vi "CameraTest.vi"() -> ()   [LabVIEW 2016]
uses:
  <vilib>/userdefined/High Color/IMAQdx.ctl
  ListboxMenu/listbox/listbox.lvclass
  ListboxMenu/listbox/listbox.lvclass/listbox.ctl
  ListboxMenu/LNK/UP/UP.lvclass
  C:/Users/ok/Desktop/camera parameters/ListboxMenu/LNK/Parent Class/Menu.lvclass
  ListboxMenu/LNK/Delete/Delete.lvclass
  ListboxMenu/LNK/Down/Down.lvclass
  <vilib>/Utility/miscctls.llb/LVRowAndColumnTypeDef.ctl
  <vilib>/Utility/miscctls.llb/LVPositionTypeDef.ctl
  <vilib>/vision/driver/NI_Vision_Acquisition_Software.lvlib
  <resource>/objmgr/imaqdx.rc
  <vilib>/ptbypt/NI_PtbyPt.lvlib
panel:
  in  "搜索相机":bool
  in  "启动相机":bool
  in  "停止相机":bool
  in  "连续获取":bool
  in  "单次获取":bool
  out "Image":T1(plugin-control)
  in  "Enum":u16(ring) items=["Off", "On"]
  in  "String":string
  in  "U32":i16
  in  "I64":i64
  in  "DBL":dbl
  in  "Bool":bool
  in  "写入参数文件":bool
  in  "读取参数文件":bool
  in  "相机参数列表":u16(ring) items=["NULL", "AcquisitionAttributes::AdvancedEthernet::BandwidthControl::DesiredPeakBandwidth", "AcquisitionAttributes::AdvancedEthernet::Controller::DestinationMode", "AcquisitionAttributes::AdvancedEthernet::Controller::DestinationMulticastAddress", "AcquisitionAttributes::AdvancedEthernet::EventParameters::MaxOutstandingEvents", "AcquisitionAttributes::AdvancedEthernet::FirewallTraversal::Enabled", "AcquisitionAttributes::AdvancedEthernet::FirewallTraversal::KeepAliveTime", "AcquisitionAttributes::AdvancedEthernet::ResendParameters::MaxResendsPerPacket", "AcquisitionAttributes::AdvancedEthernet::ResendParameters::MemoryWindowSize", "AcquisitionAttributes::AdvancedEthernet::ResendParameters::MissingPacketTimeout", "AcquisitionAttributes::AdvancedEthernet::ResendParameters::NewPacketTimeout", "AcquisitionAttributes::AdvancedEthernet::ResendParameters::ResendBatchingPercentage", "AcquisitionAttributes::AdvancedEthernet::ResendParameters::ResendResponseTimeout", "AcquisitionAttributes::AdvancedEthernet::ResendParameters::ResendThresholdPercentage", "AcquisitionAttributes::AdvancedEthernet::ResendParameters::ResendTimerResolution", "AcquisitionAttributes::AdvancedEthernet::ResendParameters::ResendsEnabled", "AcquisitionAttributes::AdvancedEthernet::TestPacketParameters::MaxTestPacketRetries", "AcquisitionAttributes::AdvancedEthernet::TestPacketParameters::TestPacketEnabled", "AcquisitionAttributes::AdvancedEthernet::TestPacketParameters::TestPacketTimeout", "AcquisitionAttributes::AdvancedGenicam::CommandTimeout", "AcquisitionAttributes::AdvancedGenicam::EventsEnabled", "AcquisitionAttributes::AdvancedGenicam::IgnoreCameraValidationErrors", "AcquisitionAttributes::Bayer::Algorithm", "AcquisitionAttributes::Bayer::GainB", "AcquisitionAttributes::Bayer::GainG", "AcquisitionAttributes::Bayer::GainR", "AcquisitionAttributes::Bayer::Pattern", "AcquisitionAttributes::ChunkDataDecoding::ChunkDataDecodingEnabled", "AcquisitionAttributes::ChunkDataDecoding::MaximumChunkCopySize", "CameraAttributes::AnalogControls::GainAuto", "CameraAttributes::AnalogControls::GainSelector", "CameraAttributes::AnalogControls::GainRaw", "CameraAttributes::AnalogControls::BlackLevelSelector", "CameraAttributes::AnalogControls::BlackLevelRaw", "CameraAttributes::AnalogControls::GammaEnable", "CameraAttributes::AnalogControls::GammaSelector", "CameraAttributes::AnalogControls::Gamma", "CameraAttributes::AnalogControls::DigitalShift", "CameraAttributes::ImageFormat::PixelFormat", "CameraAttributes::ImageFormat::ReverseX", "CameraAttributes::ImageFormat::TestImageSelector", "CameraAttributes::AOI::Width", "CameraAttributes::AOI::Height", "CameraAttributes::AOI::OffsetX", "CameraAttributes::AOI::OffsetY", "CameraAttributes::AOI::CenterX", "CameraAttributes::AOI::CenterY", "CameraAttributes::AOI::BinningHorizontal", "CameraAttributes::AOI::BinningVertical", "CameraAttributes::AcquisitionTrigger::AcquisitionMode", "CameraAttributes::AcquisitionTrigger::AcquisitionFrameCount", "CameraAttributes::AcquisitionTrigger::TriggerSelector", "CameraAttributes::AcquisitionTrigger::TriggerMode", "CameraAttributes::AcquisitionTrigger::TriggerSoftware", "CameraAttributes::AcquisitionTrigger::TriggerSource", "CameraAttributes::AcquisitionTrigger::TriggerActivation", "CameraAttributes::AcquisitionTrigger::TriggerDelayAbs", "CameraAttributes::AcquisitionTrigger::ExposureMode", "CameraAttributes::AcquisitionTrigger::ExposureAuto", "CameraAttributes::AcquisitionTrigger::ExposureTimeAbs", "CameraAttributes::AcquisitionTrigger::ExposureTimeRaw", "CameraAttributes::AcquisitionTrigger::GlobalResetReleaseModeEnable", "CameraAttributes::AcquisitionTrigger::AcquisitionFrameRateEnable", "CameraAttributes::AcquisitionTrigger::AcquisitionFrameRateAbs", "CameraAttributes::AcquisitionTrigger::AcquisitionStatusSelector", "CameraAttributes::DigitalIO::LineSelector", "CameraAttributes::DigitalIO::LineMode", "CameraAttributes::DigitalIO::LineFormat", "CameraAttributes::DigitalIO::LineSource", "CameraAttributes::DigitalIO::LineInverter", "CameraAttributes::DigitalIO::UserOutputSelector", "CameraAttributes::DigitalIO::UserOutputValue", "CameraAttributes::DigitalIO::UserOutputValueAll", "CameraAttributes::SequenceControl::SequenceEnable", "CameraAttributes::SequenceControl::SequenceControlConfiguration::SequenceAdvanceMode", "CameraAttributes::SequenceControl::SequenceSetTotalNumber", "CameraAttributes::SequenceControl::SequenceSetIndex", "CameraAttributes::SequenceControl::SequenceSetStore", "CameraAttributes::SequenceControl::SequenceSetLoad", "CameraAttributes::SequenceControl::SequenceSetExecutions", "CameraAttributes::TimerControls::TimerDelayTimebaseAbs", "CameraAttributes::TimerControls::TimerDurationTimebaseAbs", "CameraAttributes::TimerControls::TimerSelector", "CameraAttributes::TimerControls::TimerDelayAbs", "CameraAttributes::TimerControls::TimerDelayRaw", "CameraAttributes::TimerControls::TimerDurationAbs", "CameraAttributes::TimerControls::TimerDurationRaw", "CameraAttributes::TimerControls::TimerTriggerSource", "CameraAttributes::TimerControls::TimerTriggerActivation", "CameraAttributes::TimerControls::CounterSelector", "CameraAttributes::TimerControls::CounterEventSource", "CameraAttributes::TimerControls::CounterResetSource", "CameraAttributes::LUTControls::LUTSelector", "CameraAttributes::LUTControls::LUTEnable", "CameraAttributes::LUTControls::LUTIndex", "CameraAttributes::LUTControls::LUTValue", "CameraAttributes::UserDefinedValues::UserDefinedValueSelector", "CameraAttributes::UserDefinedValues::UserDefinedValue", "CameraAttributes::DeviceInformation::DeviceUserID", "CameraAttributes::ChunkDataStreams::ChunkModeActive", "CameraAttributes::EventsGeneration::EventSelector", "CameraAttributes::EventsGeneration::EventNotification", "CameraAttributes::UserSets::UserSetSelector", "CameraAttributes::UserSets::UserSetLoad", "CameraAttributes::UserSets::UserSetSave", "CameraAttributes::UserSets::UserSetDefaultSelector", "CameraAttributes::UserSets::DefaultSetSelector", "CameraAttributes::TransportLayer::GevSCFTD", "CameraAttributes::TransportLayer::GevSCBWR", "CameraAttributes::TransportLayer::GevSCBWRA", "CameraAttributes::TransportLayer::GevTimestampControlReset", "CameraAttributes::TransportLayer::GevTimestampControlLatchReset", "CameraAttributes::FileAccessControl::FileSelector", "CameraAttributes::FileAccessControl::FileOperationSelector", "CameraAttributes::FileAccessControl::FileOpenMode", "CameraAttributes::FileAccessControl::FileAccessOffset", "CameraAttributes::FileAccessControl::FileAccessLength", "CameraAttributes::FileAccessControl::FileOperationExecute", "CameraAttributes::AutoFunctions::AutoTargetValue", "CameraAttributes::AutoFunctions::AutoGainRawLowerLimit", "CameraAttributes::AutoFunctions::AutoGainRawUpperLimit", "CameraAttributes::AutoFunctions::AutoExposureTimeAbsLowerLimit", "CameraAttributes::AutoFunctions::AutoExposureTimeAbsUpperLimit", "CameraAttributes::AutoFunctions::AutoFunctionProfile", "CameraAttributes::AutoFunctions::AutoFunctionAOIs::AutoFunctionAOISelector", "CameraAttributes::AutoFunctions::AutoFunctionAOIs::AutoFunctionAOIWidth", "CameraAttributes::AutoFunctions::AutoFunctionAOIs::AutoFunctionAOIHeight", "CameraAttributes::AutoFunctions::AutoFunctionAOIs::AutoFunctionAOIOffsetX", "CameraAttributes::AutoFunctions::AutoFunctionAOIs::AutoFunctionAOIOffsetY", "CameraAttributes::AutoFunctions::AutoFunctionAOIs::AutoFunctionAOIUsageIntensity", "CameraAttributes::AutoFunctions::AutoFunctionAOIs::AutoFunctionAOIUsageWhiteBalance", "CameraAttributes::ExpertFeatureAccess::ExpertFeatureAccessSelector", "CameraAttributes::ExpertFeatureAccess::ExpertFeatureAccessKey", "AcquisitionAttributes::BitsPerPixel", "AcquisitionAttributes::ImageDecoderCopyMode", "AcquisitionAttributes::IncompleteBufferMode", "AcquisitionAttributes::OutputImageType", "AcquisitionAttributes::OverwriteMode", "AcquisitionAttributes::PacketSize", "AcquisitionAttributes::ReceiveTimestampMode", "AcquisitionAttributes::ShiftPixelBits", "AcquisitionAttributes::SwapPixelBytes", "AcquisitionAttributes::Timeout"]
  in  "添加参数":bool
  in  "写入参数":bool
  in  "获取参数值":bool
  in  "打开相机":bool
  in  "相机参数":i32(listbox)
  in  "相机列表":u16(ring) items=["acA2500-14gm:\"cam0\""]
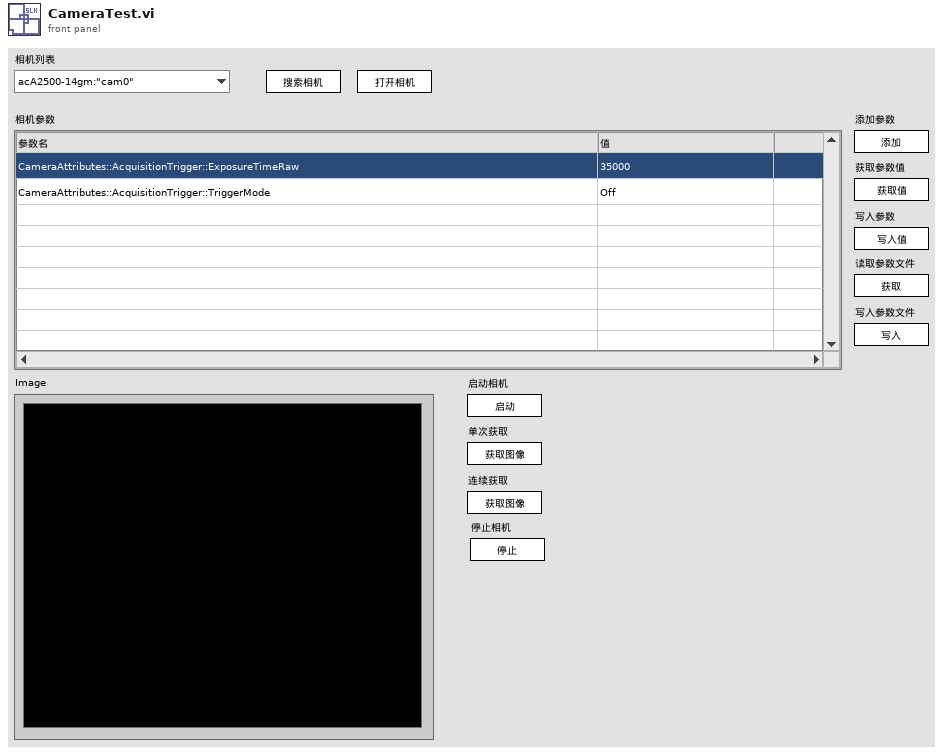
[diagram p1: front panel]
types:
  T1 = typedef "IMAQ Image.ctl" = refnum<image>
  T2 = typedef "Image Type" = u32
  T3 = typedef "IMAQdx.ctl" = refnum<k21>
  T4 = typedef "LVRowAndColumnTypeDef.ctl" = cluster{"Row":i32, "Column":i32}
  T5 = typedef "LVPositionTypeDef.ctl" = cluster{"Left":i32, "Top":i32}
  T6 = cluster{"Type":u32, "Version":u32, "Flags":u32, "SerialNumberHigh":u32, "SerialNumberLow":u32, "BusType":u32, "InterfaceName":string, "VendorName":string, "ModelName":string, "CameraFileName":string, "CameraAttributeURL":string}[]
  T7 = cluster{"Type":u32, "Version":u32, "Flags":u32, "SerialNumberHigh":u32, "SerialNumberLow":u32, "BusType":u32, "InterfaceName":string, "VendorName":string, "ModelName":string, "CameraFileName":string, "CameraAttributeURL":string}
  T8 = typedef "LVPoint32TypeDef.ctl" = cluster{"Horizontal":i32, "Vertical":i32}
  T9 = typedef "NI_Vision_Acquisition_Software.lvlib/IMAQdx Attribute Type.ctl" = enum32{"U32", "I64", "DBL", "String", "Enum", "Bool", "Command"}
  T10 = cluster{"Attribute Type":T9, "Readable":bool, "Writable":bool, "Attribute Name":string}[]
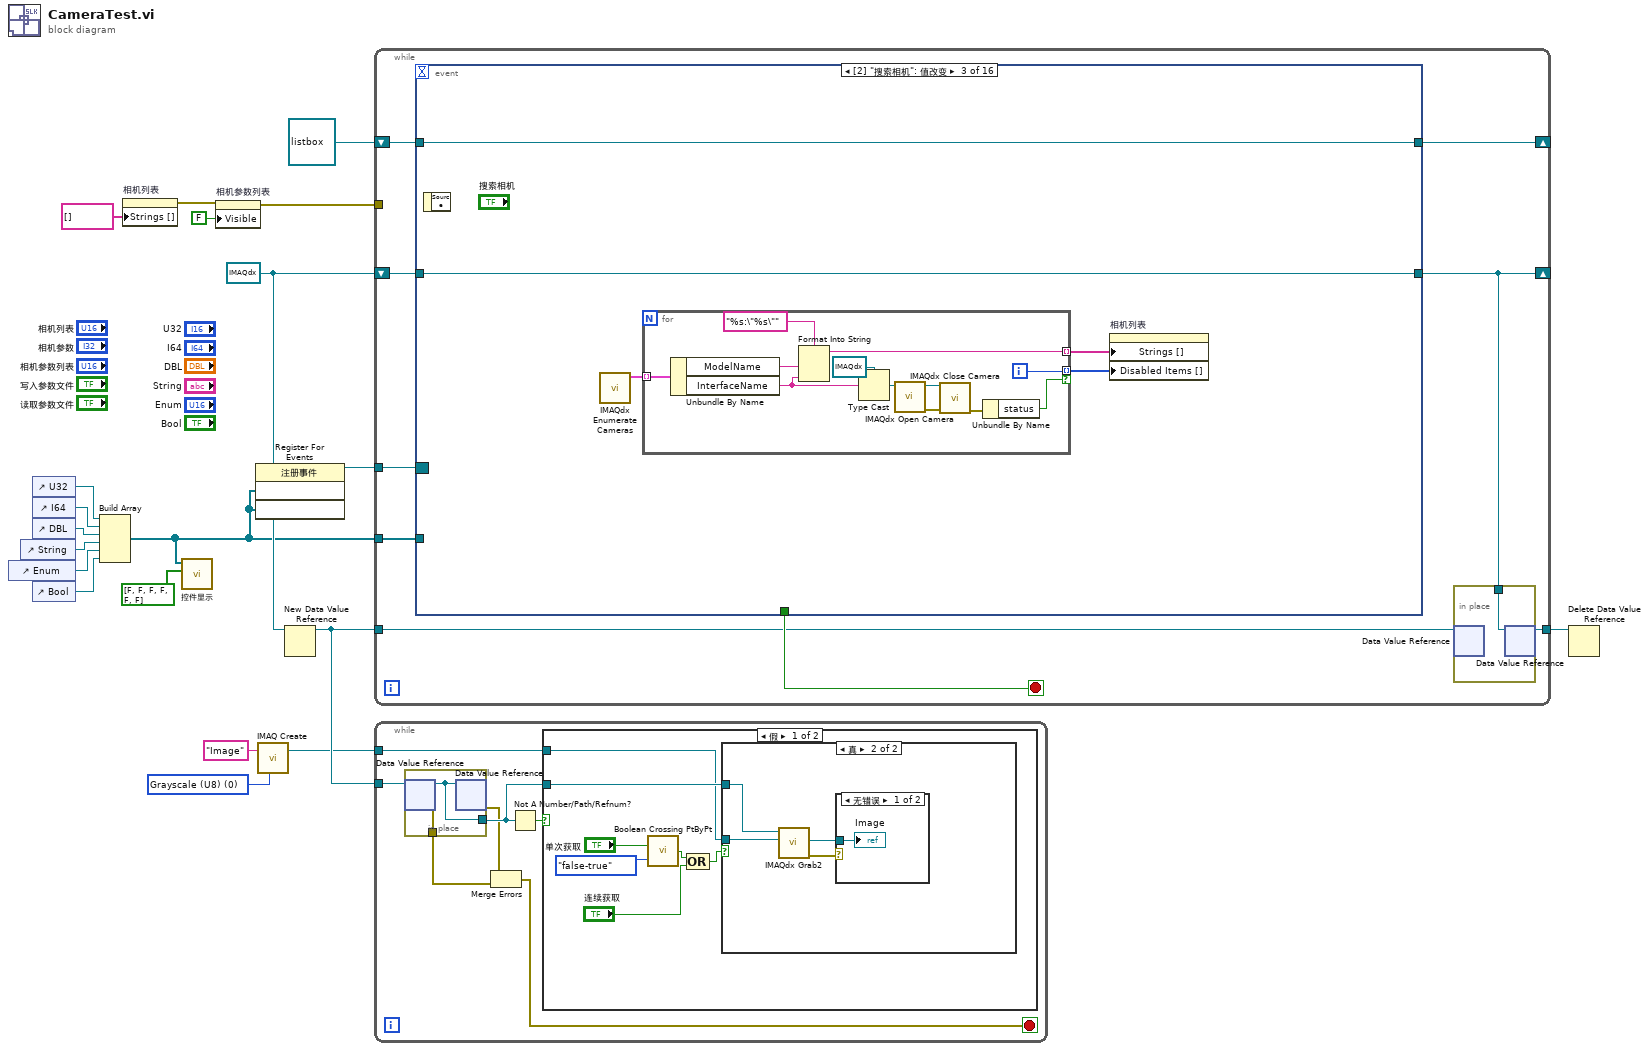
[diagram p0: block diagram]
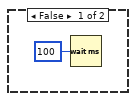
[diagram p2: hidden frame]
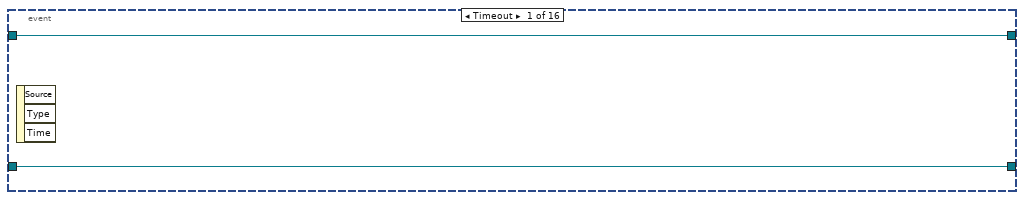
[diagram p5: hidden frame]
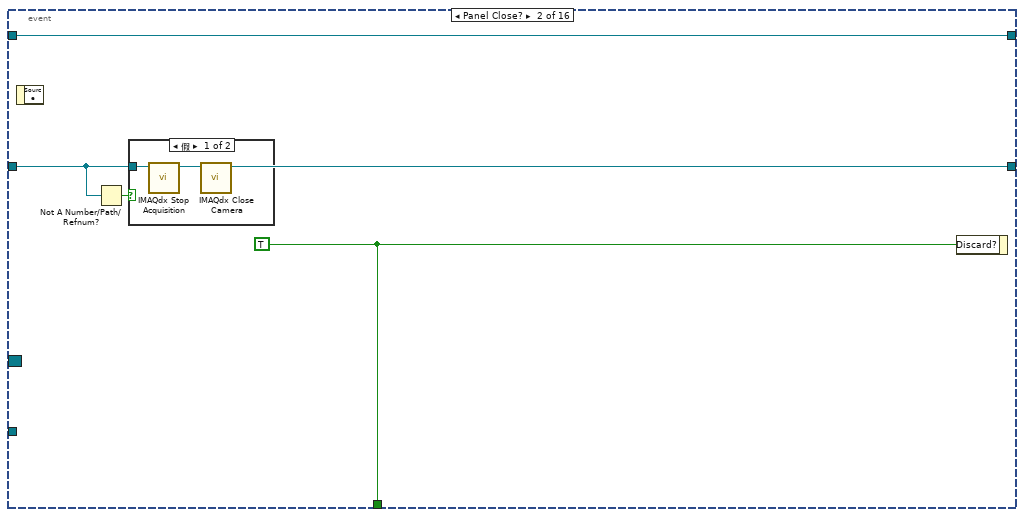
[diagram p6: hidden frame]
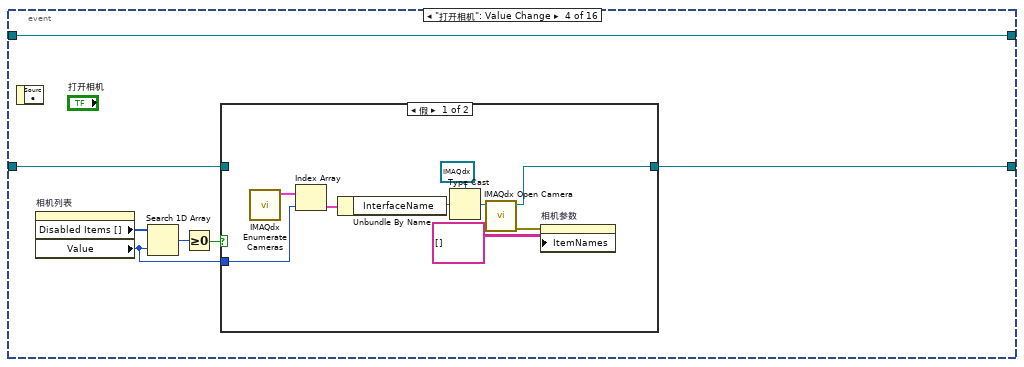
[diagram p8: hidden frame]
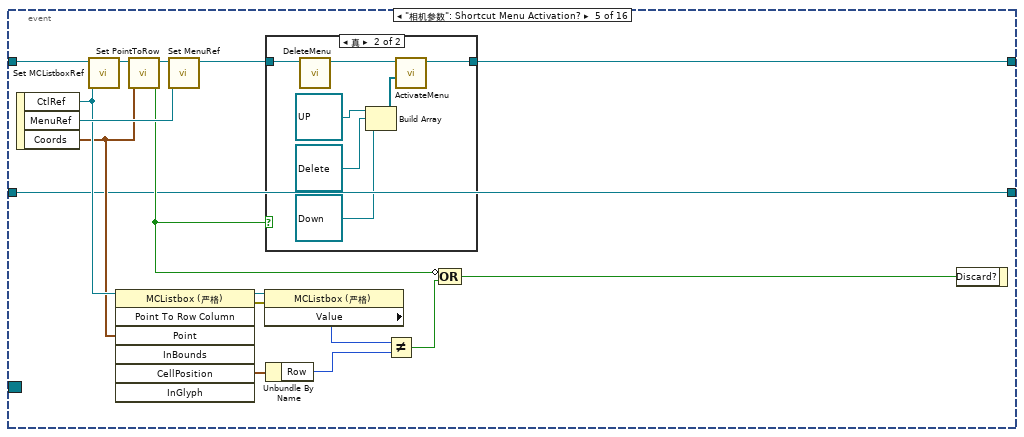
[diagram p10: hidden frame]
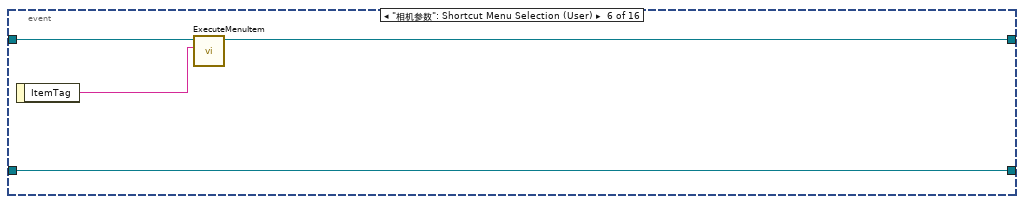
[diagram p12: hidden frame]
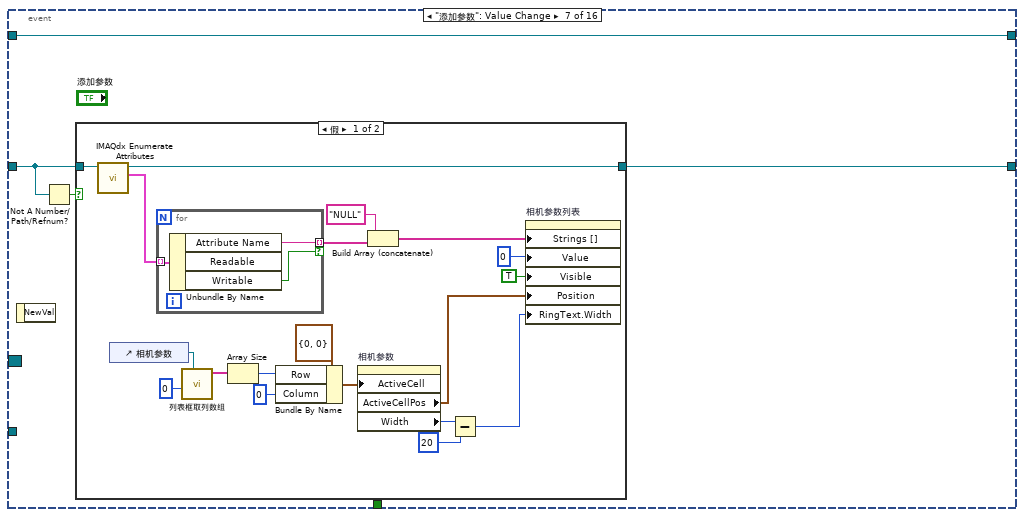
[diagram p13: hidden frame]
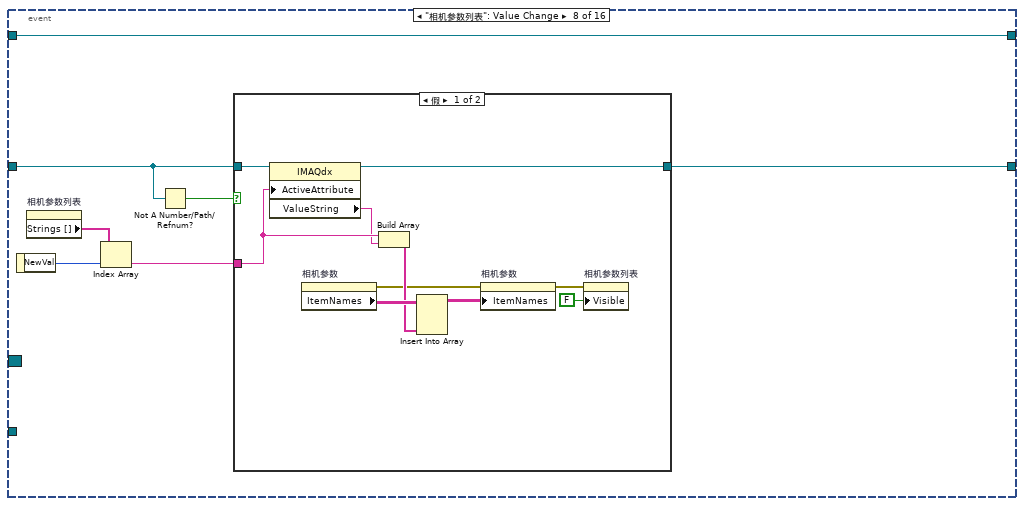
[diagram p15: hidden frame]
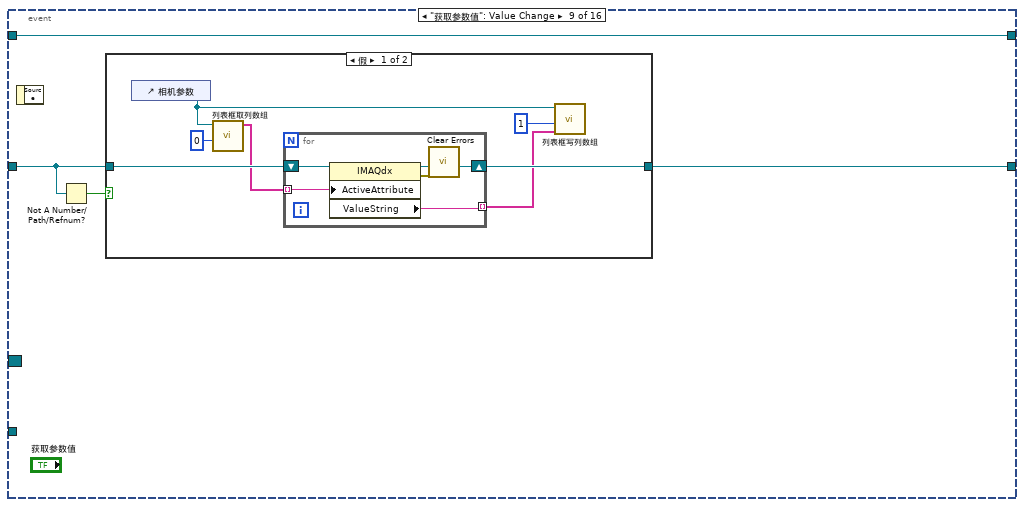
[diagram p17: hidden frame]
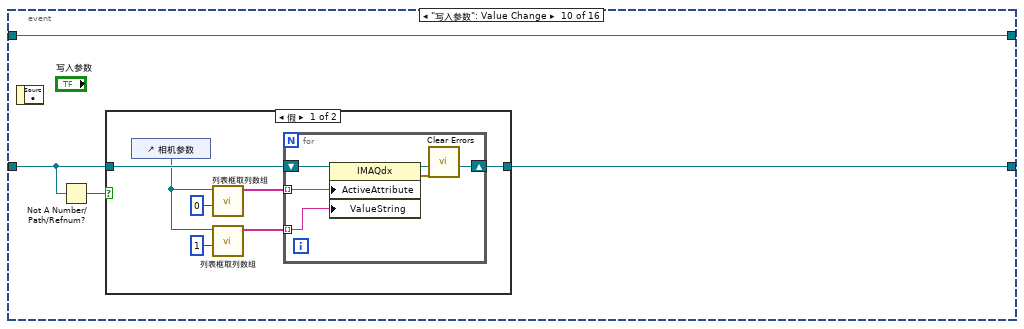
[diagram p19: hidden frame]
diagram:
  w5 = T2 0 items=["Grayscale (U8)", "Grayscale (I16)", "Grayscale (SGL)", "Complex (CSG)", "RGB (U32)", "HSL (U32)", "RGB (U64)", "Grayscale (U16)"] ("Image Type")
  w17 = T3 refnum ("Session In")
  n1 = control-ref of="Enum"() -> (w14:refnum<vi>)
  n2 = control-ref of="String"() -> (w11:refnum<vi>)
  n3 = control-ref of="U32"() -> (w16:refnum<vi>)
  n4 = control-ref of="I64"() -> (w13:refnum<vi>)
  n5 = control-ref of="DBL"() -> (w12:refnum<vi>)
  n6 = control-ref of="Bool"() -> (w15:refnum<vi>)
  n7 = Build Array(w16, w13, w12, w11, w14, w15) -> (w1:refnum<vi>[])
  n8 = property on="相机列表" class="Ring (严格)"("Strings []"=string[] [] ("字符串[]")) -> (error out=w2:errorcluster)  [unwired: 2 in, 1 out]
  n9 = call "控件显示.vi"("Visible"=bool[] [FALSE, FALSE, FALSE, FALSE, FALSE, FALSE], "Ctl"=w1) -> ()  [unwired: 10 in]
  n10 = property on="相机参数列表" class="Ring (严格)"(error in=w2, "Visible"=FALSE ("可见")) -> (error out=w18:errorcluster)  [unwired: 1 in, 1 out]
  n11 = register-events(w1, w1) -> (reference out=w9:refnum<event-registration>)  [unwired: 2 in, 1 out]
  n12 = call "IMAQ Create"("Image Name"="Image", "Image Type"=w5) -> ("New Image"=w4:T1)  [unwired: 3 in, 1 out]
  n13 = New Data Value Reference(data value=w17) -> (data value reference=w7:refnum<data-value>)  [unwired: 1 in, 1 out]
  n14 = while {
    shift-right: [w22] -> _
    shift-left: w17 -> [w28]
    shift-right: [w26] -> _
    shift-left: refnum<class "listbox.lvclass"> refnum ("listbox.lvclass") -> [w27]
    tunnel: w18 -> [_]
    tunnel: w1 -> [w25]
    tunnel: w9 -> [w24]
    tunnel: w7 -> [w23]
    tunnel: [w21] -> w8
    stop <- w29 stop-if-true
    n15 = event shown="[2] \"搜索相机\": 值改变" {
      selector: w24 -> [_ _ _ _ _ _ _ _ _ _ _ _ _ _ _ _]
      dyn-events: _ -> [_ _ _ _ _ _ _ _ _ _ _ _ _ _ _ _]
      timeout: _ -> [_ _ _ _ _ _ _ _ _ _ _ _ _ _ _ _]
      tunnel: [_ w36 _ _ _ _ _ _ _ _ _ _ _ _ _ _] -> w29
      tunnel: w28 -> [w32 w34 w42 w59 w73 w98 w104 w132 w148 w165 w182 w290 w298 w375 w378 w385]
      tunnel: [w32 w34 w42 w58 w73 w98 w103 w131 w147 w164 w181 w290 w297 w375 w377 w384] -> w22
      tunnel: w27 -> [w31 w33 w43 w57 w89 w101 w102 w135 w150 w167 w198 w291 w301 w374 w379 w386]
      tunnel: [w31 w33 w43 w57 w87 w100 w102 w135 w150 w167 w198 w291 w301 w374 w379 w386] -> w26
      tunnel: w25 -> [_ _ _ _ _ _ _ _ _ _ w183 w288 w295 _ _ _]
      event Timeout {
        n16 = event-data() -> ()  [unwired: 1 in, 3 out]
      }
      event Panel Close? {
        w36 = TRUE ("放弃？")
        n17 = event-data() -> ()  [unwired: 1 in, 1 out]
        n18 = Not A Number/Path/Refnum?(number/path/refnum=w34) -> (NaN/Path/Refnum?=w35:bool)
        n19 = case shown="假" w35 {
          tunnel: w34 -> [w38 _]
          frame False {
            n20 = call <vilib>:"IMAQdx Stop Acquisition.vi"("Session In"=w38) -> ("Session Out"=w37:T3)  [unwired: 9 in, 1 out]
            n21 = call <vilib>:"IMAQdx Close Camera.vi"("Session In"=w37) -> ()  [unwired: 10 in, 1 out]
          }
          frame True {
          }
        }
        n22 = event-data("Discard?"=w36) -> ()  [unwired: 1 in, 1 out]
      }
      event "搜索相机": Value Change {
        n23 = event-data() -> ()  [unwired: 1 in, 1 out]
        n24 = call <vilib>:"IMAQdx Enumerate Cameras.vi"() -> ("Camera Information Array"=w40:T6)  [unwired: 10 in, 1 out]
        n25 = for {
          tunnel: w40 -> [w55] mode=indexing
          tunnel: [w52] -> w39 mode=indexing
          tunnel: [w51] -> w41 mode=indexing if=w47
          i -> [w51]
          n26 = Unbundle By Name(w55) -> ("ModelName"=w54:string, "InterfaceName"=w48:string)
          n27 = Format Into String(format string="%s:\"%s\"" ("格式字符串"), w54, w48) -> (resulting string=w52:string)  [unwired: 2 in, 1 out]
          n28 = Type Cast(type=T3 refnum ("Session In"), x=w48) -> (*(type *) &x=w49:T3)
          n29 = call <vilib>:"IMAQdx Open Camera.vi"("Session In"=w49) -> ("error out"=w46:errorcluster, "Session Out"=w45:T3)  [unwired: 9 in]
          n30 = call <vilib>:"IMAQdx Close Camera.vi"("error in"=w46, "Session In"=w45) -> ("error out"=w44:errorcluster)  [unwired: 9 in]
          n31 = Unbundle By Name(w44) -> ("status"=w47:bool)
        }
        n32 = property on="相机列表" class="Ring (严格)"("Strings []"=w39, "Disabled Items []"=w41) -> ()  [unwired: 2 in, 2 out]
      }
      event "打开相机": Value Change {
        n33 = event-data() -> ()  [unwired: 1 in, 1 out]
        n34 = property on="相机列表" class="Ring (严格)"() -> ("Disabled Items []"=w62:i32[], "Value"=w56:u16)  [unwired: 2 in, 2 out]
        n35 = Search 1D Array(1D array=w62, element=w56) -> (index of element=w61:i32)  [unwired: 1 in]
        n36 = Greater Or Equal To 0?(x=w61) -> (x >= 0?=w60:bool)
        n37 = case shown="假" w60 {
          tunnel: w59 -> [_ w72]
          tunnel: [w66 w72] -> w58
          tunnel: w56 -> [w63 _]
          frame False {
            n38 = call <vilib>:"IMAQdx Enumerate Cameras.vi"() -> ("Camera Information Array"=w70:T6)  [unwired: 10 in, 1 out]
            n39 = Index Array(array=w70, index=w63) -> (element=w71:T7)
            n40 = Unbundle By Name(w71) -> ("InterfaceName"=w67:string)
            n41 = Type Cast(type=T3 refnum ("Session In"), x=w67) -> (*(type *) &x=w69:T3)
            n42 = call <vilib>:"IMAQdx Open Camera.vi"("Session In"=w69) -> ("error out"=w65:errorcluster, "Session Out"=w66:T3)  [unwired: 9 in]
            n43 = property on="相机参数" class="MCListbox (严格)"(error in=w65, "ItemNames"=string[][] [] ("项名")) -> ()  [unwired: 1 in, 2 out]
          }
          frame True {
          }
        }
      }
      event "相机参数": Shortcut Menu Activation? {
        n44 = event-data() -> ("CtlRef"=w83:refnum<vi>, "MenuRef"=w85:refnum<k9>, "Coords"=w82:T8)  [unwired: 1 in]
        n45 = call "Set MCListboxRef.vi"("MCListboxRef"=w83, "listbox in"=w89) -> ("listbox out"=w88:refnum<class "listbox.lvclass">)  [unwired: 9 in]
        n46 = invoke class="MCListbox (严格)" method="Point To Row Column"(reference=w83, "Point"=w82) -> (reference out=w80:refnum<vi>, error out=w79:errorcluster, "CellPosition"=w81:T4)  [unwired: 5 in, 4 out]
        n47 = call "Set PointToRow.vi"("坐标"=w82, "listbox 输入"=w88) -> ("边界内？"=w76:bool, "listbox 输出"=w86:refnum<class "listbox.lvclass">)  [unwired: 7 in, 1 out]
        n48 = call "Set MenuRef.vi"("MenuRef"=w85, "listbox in"=w86) -> ("listbox out"=w84:refnum<class "listbox.lvclass">)  [unwired: 9 in]
        n49 = property class="MCListbox (严格)"(reference=w80, error in=w79) -> ("Value"=w78:i32)  [unwired: 2 out]
        n50 = case shown="真" w76 {
          tunnel: w84 -> [w90 w92]
          tunnel: [w90 w93] -> w87
          frame False {
          }
          frame True {
            n51 = call "DeleteMenu.vi"("listbox 输入"=w92) -> ("listbox 输出"=w91:refnum<class "listbox.lvclass">)  [unwired: 9 in, 1 out]
            n52 = Build Array(refnum<class "UP.lvclass"> refnum ("UP.lvclass"), refnum<class "Delete.lvclass"> refnum ("Delete.lvclass"), refnum<class "Down.lvclass"> refnum ("Down.lvclass")) -> (w94:refnum<class "Menu.lvclass">[])
            n53 = call "ActivateMenu.vi"("MenuClassArray"=w94, "listbox 输入"=w91) -> ("listbox 输出"=w93:refnum<class "listbox.lvclass">)  [unwired: 8 in, 1 out]
          }
        }
        n54 = Unbundle By Name(w81) -> ("Row"=w77:i32)
        n55 = Not Equal?(x=w78, y=w77) -> (x != y?=w75:bool)
        n56 = Compound Arithmetic op=OR ("复合运算")(invert w76, w75) -> (w74:bool)
        n57 = event-data("Discard?"=w74) -> ()  [unwired: 1 in, 1 out]
      }
      event "相机参数": Shortcut Menu Selection (User) {
        n58 = event-data() -> ("ItemTag"=w99:string)  [unwired: 1 in]
        n59 = call "ExecuteMenuItem.vi"("项标识符"=w99, "listbox 输入"=w101) -> ("listbox 输出"=w100:refnum<class "listbox.lvclass">)  [unwired: 8 in, 1 out]
      }
      event "添加参数": Value Change {
        n60 = event-data() -> ()  [unwired: 1 in, 1 out]
        n61 = Not A Number/Path/Refnum?(number/path/refnum=w104) -> (NaN/Path/Refnum?=w105:bool)
        n62 = case shown="假" w105 {
          tunnel: w104 -> [w124 w128]
          tunnel: [w123 w128] -> w103
          frame False {
            n63 = call <vilib>:"IMAQdx Enumerate Attributes.vi"("Session In"=w124) -> ("Attribute Information Array"=w122:T10, "Session Out"=w123:T3)  [unwired: 8 in, 1 out]
            n64 = control-ref of="相机参数"() -> (w108:refnum<vi>)
            n65 = for {
              tunnel: w122 -> [w127] mode=indexing
              tunnel: [w126] -> w120 mode=indexing if=w125
              n66 = Unbundle By Name(w127) -> ("Attribute Name"=w126:string, "Writable"=w125:bool)  [unwired: 1 out]
            }
            n67 = call "列表框取列数组.vi"("列"=0, "引用"=w108) -> ("列数组"=w106:string[])  [unwired: 9 in]
            n68 = Array Size(array=w106) -> (size(s)=w115:i32)
            n69 = Bundle By Name(cluster=T4 {"Row"=0, "Column"=0} ("活动单元格:活动单元格"), "Row"=w115, "Column"=0) -> (w117:T4)
            n70 = property on="相机参数" class="MCListbox (严格)"("ActiveCell"=w117) -> ("ActiveCellPos"=w113:T5, "Width"=w112:u32)  [unwired: 2 in, 2 out]
            n71 = Build Array (concatenate)("NULL", w120) -> (w118:string[])
            n72 = Subtract(x=w112, y=u32 20) -> (x-y=w110:u32)
            n73 = property on="相机参数列表" class="Ring (严格)"("Strings []"=w118, "Value"=u16 0, "Visible"=TRUE ("可见"), "Position"=w113, "RingText.Width"=w110) -> ()  [unwired: 2 in, 2 out]
          }
          frame True {
          }
        }
      }
      event "相机参数列表": Value Change {
        n74 = event-data() -> ("NewVal"=w133:u16)  [unwired: 1 in]
        n75 = property on="相机参数列表" class="Ring (严格)"() -> ("Strings []"=w134:string[])  [unwired: 2 in, 2 out]
        n76 = Index Array(array=w134, index=w133) -> (element=w129:string)
        n77 = Not A Number/Path/Refnum?(number/path/refnum=w132) -> (NaN/Path/Refnum?=w130:bool)
        n78 = case shown="假" w130 {
          tunnel: w132 -> [w145 w146]
          tunnel: [w144 w146] -> w131
          tunnel: w129 -> [w143 _]
          frame False {
            n79 = property class="IMAQdx"(reference=w145, "ActiveAttribute"=w143) -> (reference out=w144:T3, "ValueString"=w142:string)  [unwired: 1 in, 1 out]
            n80 = property on="相机参数" class="MCListbox (严格)"() -> (error out=w138:errorcluster, "ItemNames"=w141:string[][])  [unwired: 2 in, 1 out]
            n81 = Build Array(w143, w142) -> (w140:string[])
            n82 = Insert Into Array(array=w141, new element=w140) -> (w139:string[][])  [unwired: 2 in]
            n83 = property on="相机参数" class="MCListbox (严格)"(error in=w138, "ItemNames"=w139) -> (error out=w137:errorcluster)  [unwired: 1 in, 1 out]
            n84 = property on="相机参数列表" class="Ring (严格)"(error in=w137, "Visible"=FALSE ("可见")) -> ()  [unwired: 1 in, 2 out]
          }
          frame True {
          }
        }
      }
      event "获取参数值": Value Change {
        n85 = event-data() -> ()  [unwired: 1 in, 1 out]
        n86 = Not A Number/Path/Refnum?(number/path/refnum=w148) -> (NaN/Path/Refnum?=w149:bool)
        n87 = case shown="假" w149 {
          tunnel: w148 -> [w156 w163]
          tunnel: [w155 w163] -> w147
          frame False {
            n88 = control-ref of="相机参数"() -> (w153:refnum<vi>)
            n89 = call "列表框取列数组.vi"("列"=0, "引用"=w153) -> ("列数组"=w154:string[])  [unwired: 9 in]
            n90 = for {
              shift-right: [w161] -> w155
              shift-left: w156 -> [w162]
              tunnel: w154 -> [w160] mode=indexing
              tunnel: [w159] -> w151 mode=indexing
              n91 = property class="IMAQdx"(reference=w162, "ActiveAttribute"=w160) -> (reference out=w161:T3, error out=w158:errorcluster, "ValueString"=w159:string)  [unwired: 1 in]
              n92 = call <vilib>:"Clear Errors.vi"("error in (no error)"=w158) -> ()  [unwired: 5 in, 2 out]
            }
            n93 = call "列表框写列数组.vi"("新元素/子数组"=w151, "列"=1, "引用"=w153) -> ()  [unwired: 9 in]
          }
          frame True {
          }
        }
      }
      event "写入参数": Value Change {
        n94 = event-data() -> ()  [unwired: 1 in, 1 out]
        n95 = Not A Number/Path/Refnum?(number/path/refnum=w165) -> (NaN/Path/Refnum?=w166:bool)
        n96 = case shown="假" w166 {
          tunnel: w165 -> [w173 w180]
          tunnel: [w172 w180] -> w164
          frame False {
            n97 = control-ref of="相机参数"() -> (w169:refnum<vi>)
            n98 = call "列表框取列数组.vi"("列"=0, "引用"=w169) -> ("列数组"=w171:string[])  [unwired: 9 in]
            n99 = call "列表框取列数组.vi"("列"=1, "引用"=w169) -> ("列数组"=w168:string[])  [unwired: 9 in]
            n100 = for {
              shift-right: [w178] -> w172
              shift-left: w173 -> [w179]
              tunnel: w171 -> [w177] mode=indexing
              tunnel: w168 -> [w175] mode=indexing
              n101 = property class="IMAQdx"(reference=w179, "ActiveAttribute"=w177, "ValueString"=w175) -> (reference out=w178:T3, error out=w176:errorcluster)  [unwired: 1 in]
              n102 = call <vilib>:"Clear Errors.vi"("error in (no error)"=w176) -> ()  [unwired: 5 in, 2 out]
            }
          }
          frame True {
          }
        }
      }
      event "相机参数": Mouse Down {
        n103 = event-data() -> ("CtlRef"=w193:refnum<vi>, "Coords"=w192:T8)  [unwired: 1 in]
        n104 = invoke class="MCListbox (严格)" method="Point To Row Column"(reference=w193, "Point"=w192) -> (reference out=w196:refnum<vi>, error out=w195:errorcluster, "CellPosition"=w197:T4)  [unwired: 5 in, 4 out]
        n105 = property class="MCListbox (严格)"(reference=w196, error in=w195) -> (reference out=w189:refnum<vi>, "Value"=w188:i32)  [unwired: 1 out]
        n106 = Unbundle By Name(w197) -> ("Row"=w194:i32, "Column"=w191:i32)
        n107 = Equal?(x=w188, y=w194) -> (x = y?=w186:bool)
        n108 = Equal?(x=w191, y=1) -> (x = y?=w185:bool)
        n109 = Not A Number/Path/Refnum?(number/path/refnum=w182) -> (NaN/Path/Refnum?=w187:bool)
        n110 = Compound Arithmetic op=AND ("复合运算")(invert w187, w186, w185) -> (w184:bool)
        n111 = case shown="真" w184 {
          tunnel: w189 -> [_ w213]
          tunnel: w188 -> [_ w212]
          tunnel: w182 -> [w201 w216]
          tunnel: w183 -> [w199 w205]
          tunnel: [w201 w203] -> w181
          frame False {
            n112 = call "控件显示.vi"("Visible"=bool[] [FALSE, FALSE, FALSE, FALSE, FALSE, FALSE], "Ctl"=w199) -> ()  [unwired: 10 in]
          }
          frame True {
            n113 = Bundle By Name(cluster=T4 {"Row"=0, "Column"=0} ("活动单元格:活动单元格"), "Row"=w212, "Column"=1) -> (w215:T4)
            n114 = call "列表框取列数组.vi"("列"=0, "引用"=w213) -> ("列数组"=w217:string[])  [unwired: 9 in]
            n115 = Index Array(array=w217, index=w212) -> (element=w206:string)
            n116 = property on="属性节点" class="MCListbox (严格)"(reference=w213, "ActiveCell"=w215, "Height"=u32 24 ("活动单元格:单元格大小:高度")) -> ("ActiveCellPos"=w210:T5)  [unwired: 1 in, 2 out]
            n117 = property class="IMAQdx"(reference=w216, "ActiveAttribute"=w206) -> (reference out=w207:T3, "Type"=w208:u32)  [unwired: 1 in, 1 out]
            n118 = Add(x=w210, y=T5 {"Left"=50, "Top"=0}) -> (x+y=w204:T5)
            n119 = case shown="2" w208 {
              selector: w208 -> [w227 w238 w250 w261 w273 w284 _]
              tunnel: w207 -> [w229 w240 w252 w263 w275 w286 w287]
              tunnel: w206 -> [w228 w239 w251 w262 w274 w285 _]
              tunnel: w205 -> [w220 w231 w244 w256 w269 w280 _]
              tunnel: w204 -> [w222 w235 w247 w258 w270 w281 _]
              tunnel: [w219 w230 w242 w253 w264 w276 w287] -> w203
              frame 0 {
                n120 = property class="IMAQdx"(reference=w229, "ActiveAttribute"=w228) -> (reference out=w219:T3, "ValueU32"=w224:u32)  [unwired: 1 in, 1 out]
                n121 = Index Array(array=w220, index=w227) -> (element=w226:refnum<vi>)
                n122 = To More Specific Class(target class=refnum<vi> refnum ("U32"), reference=w226) -> (specific class reference=w223:refnum<vi>)  [unwired: 1 in, 1 out]
                n123 = property class="DigNum (严格)"(reference=w223, "Value"=w224, "Position"=w222) -> ()  [unwired: 1 in, 2 out]
                n124 = call "控件显示.vi"("Visible"=bool[] [TRUE, FALSE, FALSE, FALSE, FALSE, FALSE], "Ctl"=w220) -> ()  [unwired: 10 in]
              }
              frame 1 {
                n125 = property class="IMAQdx"(reference=w240, "ActiveAttribute"=w239) -> (reference out=w230:T3, "ValueI64"=w233:i64)  [unwired: 1 in, 1 out]
                n126 = Index Array(array=w231, index=w238) -> (element=w237:refnum<vi>)
                n127 = To More Specific Class(target class=refnum<vi> refnum ("I64"), reference=w237) -> (specific class reference=w236:refnum<vi>)  [unwired: 1 in, 1 out]
                n128 = property class="DigNum (严格)"(reference=w236, "Value"=w233, "Position"=w235) -> ()  [unwired: 1 in, 2 out]
                n129 = call "控件显示.vi"("Visible"=bool[] [FALSE, TRUE, FALSE, FALSE, FALSE, FALSE], "Ctl"=w231) -> ()  [unwired: 10 in]
              }
              frame 2 {
                n130 = property class="IMAQdx"(reference=w252, "ActiveAttribute"=w251) -> (reference out=w242:T3, "ValueDBL"=w246:dbl)  [unwired: 1 in, 1 out]
                n131 = Index Array(array=w244, index=w250) -> (element=w249:refnum<vi>)
                n132 = To More Specific Class(target class=refnum<vi> refnum ("DBL"), reference=w249) -> (specific class reference=w248:refnum<vi>)  [unwired: 1 in, 1 out]
                n133 = property class="DigNum (严格)"(reference=w248, "Value"=w246, "Position"=w247, "Key Focus"=TRUE ("键选中")) -> ()  [unwired: 1 in, 2 out]
                n134 = call "控件显示.vi"("Visible"=bool[] [FALSE, FALSE, TRUE, FALSE, FALSE, FALSE], "Ctl"=w244) -> ()  [unwired: 10 in]
              }
              frame 3 {
                n135 = property class="IMAQdx"(reference=w263, "ActiveAttribute"=w262) -> (reference out=w253:T3, "ValueString"=w257:string)  [unwired: 1 in, 1 out]
                n136 = Index Array(array=w256, index=w261) -> (element=w260:refnum<vi>)
                n137 = To More Specific Class(target class=refnum<vi> refnum ("String"), reference=w260) -> (specific class reference=w259:refnum<vi>)  [unwired: 1 in, 1 out]
                n138 = property class="Str"(reference=w259, "Value"=w257, "Position"=w258) -> ()  [unwired: 1 in, 2 out]
                n139 = call "控件显示.vi"("Visible"=bool[] [FALSE, FALSE, FALSE, TRUE, FALSE, FALSE], "Ctl"=w256) -> ()  [unwired: 10 in]
              }
              frame 4 {
                n140 = property class="IMAQdx"(reference=w275, "ActiveAttribute"=w274) -> (reference out=w264:T3, "EnumStrings[]"=w266:string[], "ValueU32"=w265:u32)  [unwired: 1 in, 1 out]
                n141 = Index Array(array=w269, index=w273) -> (element=w272:refnum<vi>)
                n142 = To More Specific Class(target class=refnum<vi> refnum ("Enum"), reference=w272) -> (specific class reference=w271:refnum<vi>)  [unwired: 1 in, 1 out]
                n143 = property class="Ring (严格)"(reference=w271, "Strings []"=w266, "Position"=w270, "Value"=w265) -> ()  [unwired: 1 in, 2 out]
                n144 = call "控件显示.vi"("Visible"=bool[] [FALSE, FALSE, FALSE, FALSE, TRUE, FALSE], "Ctl"=w269) -> ()  [unwired: 10 in]
              }
              frame 5 {
                n145 = property class="IMAQdx"(reference=w286, "ActiveAttribute"=w285) -> (reference out=w276:T3, "ValueBool"=w277:bool)  [unwired: 1 in, 1 out]
                n146 = Index Array(array=w280, index=w284) -> (element=w283:refnum<vi>)
                n147 = To More Specific Class(target class=refnum<vi> refnum ("Bool"), reference=w283) -> (specific class reference=w282:refnum<vi>)  [unwired: 1 in, 1 out]
                n148 = property class="Bool (严格)"(reference=w282, "Value"=w277, "Position"=w281) -> ()  [unwired: 1 in, 2 out]
                n149 = call "控件显示.vi"("Visible"=bool[] [FALSE, FALSE, FALSE, FALSE, FALSE, TRUE], "Ctl"=w280) -> ()  [unwired: 10 in]
              }
              frame 6, Default {
              }
            }
          }
        }
      }
      event Mouse Leave {
        n150 = event-data() -> ()  [unwired: 1 in, 4 out]
        n151 = call "控件显示.vi"("Visible"=bool[] [FALSE, FALSE, FALSE, FALSE, FALSE, FALSE], "Ctl"=w288) -> ()  [unwired: 10 in]
      }
      event Value Change {
        n152 = event-data() -> ("CtlRef"=w294:refnum<vi>)  [unwired: 1 in]
        n153 = control-ref of="相机参数"() -> (w296:refnum<vi>)
        n154 = property class="MCListbox (严格)"(reference=w296) -> (reference out=w300:refnum<vi>, "Value"=w299:i32)  [unwired: 1 in, 1 out]
        n155 = Search 1D Array(1D array=w295, element=w294) -> (index of element=w293:i32)  [unwired: 1 in]
        n156 = Not A Number/Path/Refnum?(number/path/refnum=w298) -> (NaN/Path/Refnum?=w292:bool)
        n157 = case shown="假" w292 {
          tunnel: w300 -> [w314 _]
          tunnel: w299 -> [w306 _]
          tunnel: w298 -> [w315 w373]
          tunnel: w295 -> [w311 _]
          tunnel: [w309 w373] -> w297
          tunnel: w293 -> [w313 _]
          frame False {
            w303 = 1 ("列")
            n158 = call "列表框取列数组.vi"("列"=0, "引用"=w314) -> ("列数组"=w316:string[])  [unwired: 9 in]
            n159 = call "控件显示.vi"("Visible"=bool[] [FALSE, FALSE, FALSE, FALSE, FALSE, FALSE], "Ctl"=w311) -> ()  [unwired: 10 in]
            n160 = Index Array(array=w316, index=w306) -> (element=w308:string)
            n161 = case shown="1" w313 {
              selector: w313 -> [w325 w334 w343 w352 w361 w370 _]
              tunnel: w315 -> [w320 w330 w339 w348 w357 w366 w372]
              tunnel: w308 -> [w326 w335 w344 w353 w362 w371 _]
              tunnel: w311 -> [w321 w331 w340 w349 w358 w367 _]
              tunnel: [w319 w329 w338 w347 w356 w365 w372] -> w310
              frame 0 {
                n162 = Index Array(array=w321, index=w325) -> (element=w324:refnum<vi>)
                n163 = To More Specific Class(target class=refnum<vi> refnum ("U32"), reference=w324) -> (specific class reference=w322:refnum<vi>)  [unwired: 1 in, 1 out]
                n164 = property class="DigNum (严格)"(reference=w322) -> ("Value"=w318:i16)  [unwired: 1 in, 2 out]
                n165 = property class="IMAQdx"(reference=w320, "ActiveAttribute"=w326, "ValueU32"=w318) -> (reference out=w319:T3)  [unwired: 1 in, 1 out]
              }
              frame 1 {
                n166 = Index Array(array=w331, index=w334) -> (element=w333:refnum<vi>)
                n167 = To More Specific Class(target class=refnum<vi> refnum ("I64"), reference=w333) -> (specific class reference=w332:refnum<vi>)  [unwired: 1 in, 1 out]
                n168 = property class="DigNum (严格)"(reference=w332) -> ("Value"=w328:i64)  [unwired: 1 in, 2 out]
                n169 = property class="IMAQdx"(reference=w330, "ActiveAttribute"=w335, "ValueI64"=w328) -> (reference out=w329:T3)  [unwired: 1 in, 1 out]
              }
              frame 2 {
                n170 = Index Array(array=w340, index=w343) -> (element=w342:refnum<vi>)
                n171 = To More Specific Class(target class=refnum<vi> refnum ("DBL"), reference=w342) -> (specific class reference=w341:refnum<vi>)  [unwired: 1 in, 1 out]
                n172 = property class="DigNum (严格)"(reference=w341) -> ("Value"=w337:dbl)  [unwired: 1 in, 2 out]
                n173 = property class="IMAQdx"(reference=w339, "ActiveAttribute"=w344, "ValueDBL"=w337) -> (reference out=w338:T3)  [unwired: 1 in, 1 out]
              }
              frame 3 {
                n174 = Index Array(array=w349, index=w352) -> (element=w351:refnum<vi>)
                n175 = To More Specific Class(target class=refnum<vi> refnum ("String"), reference=w351) -> (specific class reference=w350:refnum<vi>)  [unwired: 1 in, 1 out]
                n176 = property class="Str"(reference=w350) -> ("Value"=w346:string)  [unwired: 1 in, 2 out]
                n177 = property class="IMAQdx"(reference=w348, "ActiveAttribute"=w353, "ValueString"=w346) -> (reference out=w347:T3)  [unwired: 1 in, 1 out]
              }
              frame 4 {
                n178 = Index Array(array=w358, index=w361) -> (element=w360:refnum<vi>)
                n179 = To More Specific Class(target class=refnum<vi> refnum ("Enum"), reference=w360) -> (specific class reference=w359:refnum<vi>)  [unwired: 1 in, 1 out]
                n180 = property class="Ring (严格)"(reference=w359) -> ("Value"=w355:u16)  [unwired: 1 in, 2 out]
                n181 = property class="IMAQdx"(reference=w357, "ActiveAttribute"=w362, "ValueU32"=w355) -> (reference out=w356:T3)  [unwired: 1 in, 1 out]
              }
              frame 5 {
                n182 = Index Array(array=w367, index=w370) -> (element=w369:refnum<vi>)
                n183 = To More Specific Class(target class=refnum<vi> refnum ("Bool"), reference=w369) -> (specific class reference=w368:refnum<vi>)  [unwired: 1 in, 1 out]
                n184 = property class="Bool (严格)"(reference=w368) -> ("Value"=w364:bool)  [unwired: 1 in, 2 out]
                n185 = property class="IMAQdx"(reference=w366, "ActiveAttribute"=w371, "ValueBool"=w364) -> (reference out=w365:T3)  [unwired: 1 in, 1 out]
              }
              frame 6, Default {
              }
            }
            n186 = control-ref of="相机参数"() -> (w305:refnum<vi>)
            n187 = property class="IMAQdx"(reference=w310, "ActiveAttribute"=w308) -> (reference out=w309:T3, "ValueString"=w302:string)  [unwired: 1 in, 1 out]
            n188 = call "列表框取列数组.vi"("列"=w303, "引用"=w305) -> ("列数组"=w307:string[])  [unwired: 9 in]
            n189 = Replace Array Subset(array=w307, new element=w302, index=w306) -> (w304:string[])
            n190 = call "列表框写列数组.vi"("新元素/子数组"=w304, "列"=w303, "引用"=w305) -> ()  [unwired: 9 in]
          }
          frame True {
          }
        }
      }
      event "相机参数": Value Change {
        n191 = event-data() -> ()  [unwired: 1 in, 6 out]
      }
      event "启动相机": Value Change {
        n192 = event-data() -> ()  [unwired: 1 in, 6 out]
        n193 = Not A Number/Path/Refnum?(number/path/refnum=w378) -> (NaN/Path/Refnum?=w376:bool)
        n194 = case shown="假" w376 {
          tunnel: w378 -> [w381 w382]
          tunnel: [w380 w382] -> w377
          frame False {
            n195 = call <vilib>:"IMAQdx Configure Grab.vi"("Session In"=w381) -> ("Session Out"=w380:T3)  [unwired: 9 in, 1 out]
          }
          frame True {
          }
        }
      }
      event "停止相机": Value Change {
        n196 = event-data() -> ()  [unwired: 1 in, 6 out]
        n197 = Not A Number/Path/Refnum?(number/path/refnum=w385) -> (NaN/Path/Refnum?=w383:bool)
        n198 = case shown="假" w383 {
          tunnel: w385 -> [w389 w390]
          tunnel: [w388 w390] -> w384
          frame False {
            n199 = call <vilib>:"IMAQdx Stop Acquisition.vi"("Session In"=w389) -> ("Session Out"=w388:T3)  [unwired: 9 in, 1 out]
            n200 = local write "连续获取"(FALSE ("连续获取")) -> ()
          }
          frame True {
          }
        }
      }
    }
    n201 = in-place {
      in-place-border: w22 -> [w30]
      n202 = in-place-dvr #1(w23) -> ()  [unwired: 2 out]
      n203 = in-place-dvr #1(w30) -> (w21:refnum<data-value>)  [unwired: 1 out]
    }
  }
  n204 = while {
    tunnel: w7 -> [w397]
    tunnel: w4 -> [w394]
    stop <- w391 stop-if-true
    n205 = in-place {
      in-place-border: [w412] -> w395
      in-place-border: [w411] -> w392
      n206 = in-place-dvr #2(w397) -> (w412:T3, w411:errorcluster)
      n207 = in-place-dvr #2(w412) -> (w393:errorcluster)  [unwired: 1 out]
    }
    n208 = Merge Errors(w393, w392) -> (w391:errorcluster)
    n209 = Not A Number/Path/Refnum?(number/path/refnum=w395) -> (NaN/Path/Refnum?=w396:bool)
    n210 = case shown="假" w396 {
      tunnel: w395 -> [w402 _]
      tunnel: w394 -> [w401 _]
      frame False {
        n211 = call <vilib>:"Boolean Crossing PtByPt.vi"("direction"=enum16{"either", "false-true", "true-false"}."false-true", "input"="单次获取") -> ("crossing"=w400:bool)  [unwired: 1 in]
        n212 = Compound Arithmetic op=OR ("复合运算")(w400, "连续获取") -> (w398:bool)
        n213 = case shown="真" w398 {
          tunnel: w402 -> [_ w409]
          tunnel: w401 -> [_ w408]
          frame False {
            n214 = Wait (ms)(milliseconds to wait=u32 100 ("等待时间（毫秒）")) -> ()  [unwired: 1 out]
          }
          frame True {
            n215 = call <vilib>:"IMAQdx Grab2.vi"("Image In"=w408, "Session In"=w409) -> ("error out"=w406:errorcluster, "Image Out"=w407:T1)  [unwired: 6 in, 2 out]
            n216 = case shown="无错误" w406 {
              tunnel: w407 -> [w410 _]
              frame No Error {
                "Image" <- w410
              }
              frame Error {
              }
            }
          }
        }
      }
      frame True {
      }
    }
  }
  n217 = Delete Data Value Reference(data value reference=w8) -> ()  [unwired: 1 in, 2 out]
